vi "Write ini.vi"   [LabVIEW 2016]
uses:
  <vilib>/Utility/config.llb/Write Key (String).vi
  <vilib>/Utility/config.llb/NI_LVConfig.lvlib
types:
  T1 = typedef "NI_LVConfig.lvlib/Config Data RefNum.ctl" = refnum<k1>
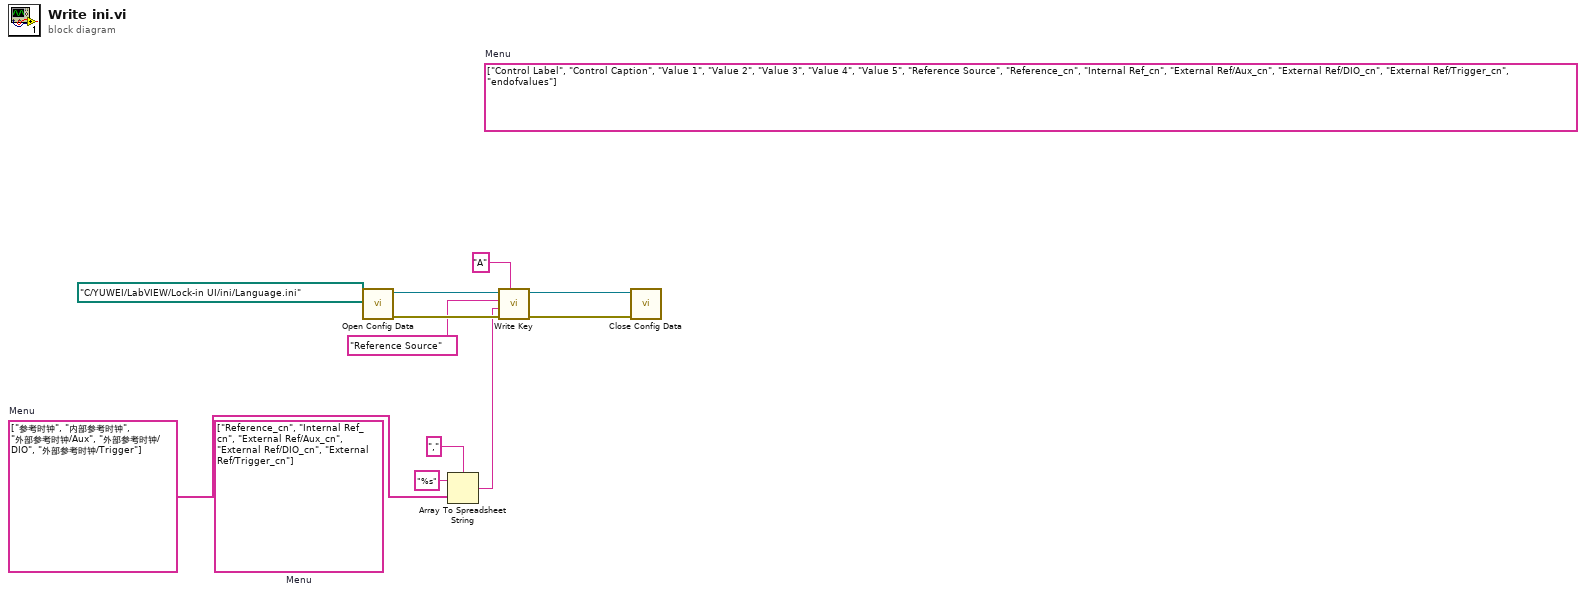
[diagram p0: block diagram]
diagram:
  w1 = string[] ["参考时钟", "内部参考时钟", "外部参考时钟/Aux", "外部参考时钟/DIO", "外部参考时钟/Trigger"]  # Menu
  (unwired) string[] ["Reference_cn", "Internal Ref_cn", "External Ref/Aux_cn", "External Ref/DIO_cn", "External Ref/Trigger_cn"]  # Menu
  (unwired) string[][] [["Control Label", "Control Caption", "Value 1", "Value 2", "Value 3", "Value 4", "Value 5"], ["Reference Source", "Reference_cn", "Internal Ref_cn", "External Ref/Aux_cn", "External Ref/DIO_cn", "External Ref/Trigger_cn", "endofvalues"]]  # Menu
  n1 = call <vilib>:"Open Config Data.vi"("configuration file path"=path "C:/YUWEI/LabVIEW/Lock-in UI/ini/Language.ini") -> ("error out"=w10:errorcluster, "refnum"=w11:T1)  [unwired: 8 in, 1 out]
  n2 = Array To Spreadsheet String(delimiter (Tab)=",", array=w1, 3:"%s" ("format string")) -> (spreadsheet string=w3:string)
  n3 = call-poly <vilib>:"Write Key.vi"("section"="A", "error in (no error)"=w10, "value"=w3, "key"="Reference Source", "refnum"=w11) -> ("error out"=w9:errorcluster, "refnum out"=w8:T1)  [unwired: 4 in, 1 out]
  n4 = call <vilib>:"Close Config Data.vi"("error in (no error)"=w9, "refnum"=w8) -> ()  [unwired: 8 in, 2 out]
